vi "Test_StartMessageCycle_ReleaseNotifier_CycleStops.vi"(8 "error in (no error)":errorcluster, 11 "TestCase in":refnum<class "TestMessageCycle.lvclass">) -> (0 "error out":errorcluster, 3 "TestCase out":refnum<class "TestMessageCycle.lvclass">)   [LabVIEW 2017, in "TestMessageCycle.lvclass"]
uses:
  TestMessageCycle.lvclass
  <vilib>/ActorFramework/Message/Message.lvclass
  Source/MessageCycle/MessageCycle.lvclass/MessageCycle.ctl
  <vilib>/ActorFramework/Message Enqueuer/Message Enqueuer.lvclass/Message Enqueuer.ctl
  cea1d73f-f580-4a5c-bd1b-22283d1460f9.vi
  <vilib>/ActorFramework/Message Enqueuer/Enqueue.vi
  Doubles/ActorCountsMessageCycles/ActorCountsMessageCycles.lvclass
  C:/Program Files (x86)/National Instruments/LabVIEW 2017/vi.lib/ActorFramework/Actor/Actor.lvclass
  Source/MessageCycle/MessageCycle.lvclass
  C:/Program Files (x86)/National Instruments/LabVIEW 2017/vi.lib/ActorFramework/Message/Message.lvclass
  <vilib>/ActorFramework/Stop Msg/Stop Msg.lvclass
  Source/MessageCycle/Launch Deferred Timeout Notifier.vi
  <vilib>/ActorFramework/Message Priority Queue/Priority Enqueue.vi
  <vilib>/ActorFramework/Actor/Actor.lvclass
panel:
  out "Cyclic Messages Received":u32
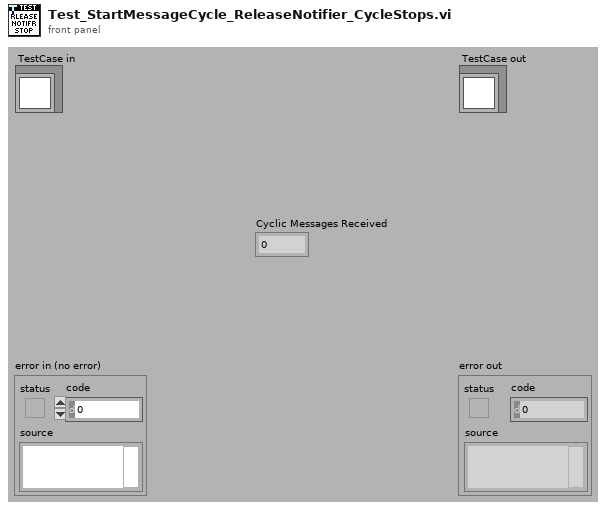
[diagram p1: front panel]
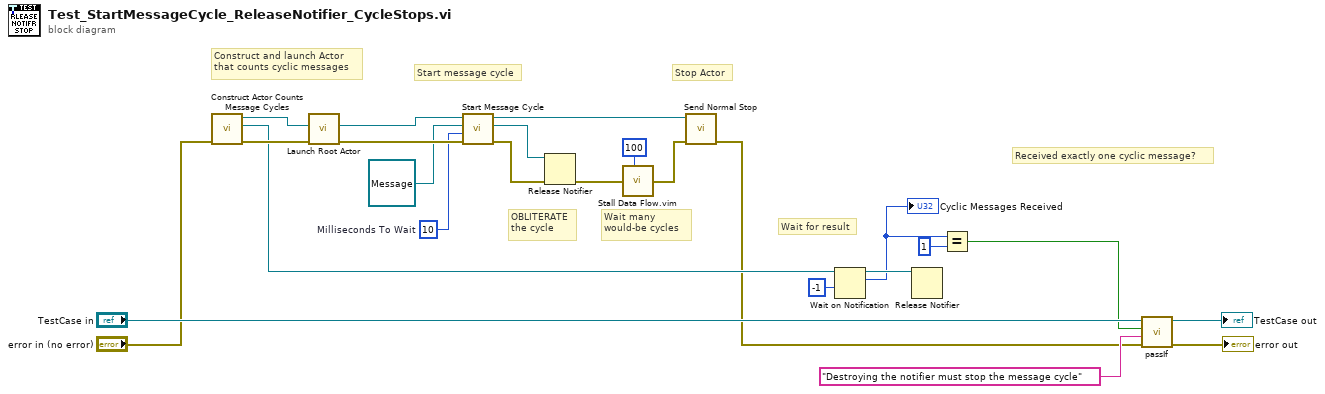
[diagram p0: block diagram]
diagram:
  w20 = 10  # Milliseconds To Wait
  # "Wait many\nwould-be cycles"
  # "OBLITERATE\nthe cycle"
  # "Wait for result"
  # "Stop Actor"
  # "Start message cycle"
  # "Received exactly one cyclic message?"
  # "Construct and launch Actor\nthat counts cyclic messages"
  n1 = call "Construct Actor Counts Message Cycles.vi"("error in (no error)"="error in (no error)") -> ("error out"=w13:errorcluster, "Final Count"=w12:refnum<notifier>, "ActorCountsMessageCycles"=w15:refnum<class "ActorCountsMessageCycles.lvclass">)  [unwired: 8 in]
  n2 = call <vilib>:"Launch Root Actor.vi"("error in (no error)"=w13, "Actor"=w15) -> ("error out"=w24:errorcluster, "Actor's Enqueuer"=w19:refnum<class "Message Enqueuer.lvclass">)  [unwired: 8 in]
  n3 = call "Start Message Cycle.vi"("error in (no error)"=w24, "Inter-Message Wait [ms] (0)"=w20, "Message"=refnum<class "Message.lvclass"> refnum, "Message Enqueuer"=w19) -> ("error out"=w5:errorcluster, "Message Cycle Notifier"=w6:refnum<notifier>, "Message Enqueuer out"=w18:refnum<class "Message Enqueuer.lvclass">)  [unwired: 5 in]
  n4 = Release Notifier(notifier=w6, error in (no error)=w5) -> (error out=w4:errorcluster)  [unwired: 1 in, 2 out]
  n5 = call "Stall Data Flow.vim"("value in"=w4, "milliseconds to wait"=u32 100) -> ("value out"=w3:errorcluster)  [unwired: 1 out]
  n6 = call <vilib>:"Send Normal Stop.vi"("error in (no error)"=w3, "Message Enqueuer"=w18) -> ("error out"=w9:errorcluster)  [unwired: 9 in]
  n7 = Wait on Notification(notifier=w12, timeout in ms (-1)=-1) -> (notifier out=w10:refnum<notifier>, notification=w8:u32)  [unwired: 2 in, 2 out]
  "Cyclic Messages Received" <- w8
  n8 = Release Notifier(notifier=w10) -> ()  [unwired: 2 in, 3 out]
  n9 = Equal?(x=w8, y=u32 1) -> (x = y?=w17:bool)
  n10 = call-dynamic "passIf.vi"("error in (no error)"=w9, "message (\"\")"="Destroying the notifier must stop the message cycle" ("message (\"\")"), "pass"=w17, "TestCase in"="TestCase in") -> ("error out"=→"error out":errorcluster, "TestCase out"=→"TestCase out":refnum<class "TestMessageCycle.lvclass">)  [unwired: 6 in]
